vi "UDP Data Link - Action VIs - ActionVIOnSave.vi"(8 "error in (no error)":errorcluster, 11 "Device Item Ref in":T1 format="%.0x") -> (0 "error out":errorcluster, 3 "Device Item Ref out":T1 format="%.0x")   [LabVIEW 2015, in "UDP-Custom-Device System Explorer.lvlib"]
uses:
  UDP-Custom-Device System Explorer.lvlib
  <vilib>/NI Veristand/Custom Device API/Custom Device Item Ref.ctl
  Shared/Constants.vi
  <vilib>/NI Veristand/Custom Device API/Get Item Property (Boolean).vi
  <vilib>/NI Veristand/Custom Device API/Get Item Property (Path).vi
  <vilib>/NI VeriStand/Custom Device API/Custom Device API.lvlib
  Shared/UDP-Custom-Device Shared.lvlib
  <vilib>/NI VeriStand/Custom Device Tools/Custom Device Utility Library/Custom Device Utility Library.lvlib
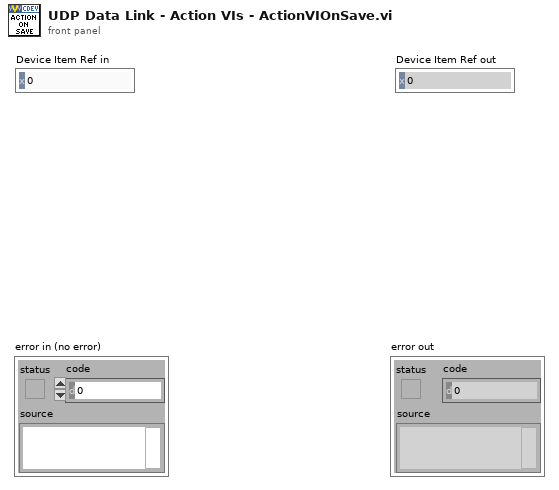
[diagram p1: front panel]
types:
  T1 = typedef "Custom Device API.lvlib/Custom Device Item Ref.ctl" = u64
  T2 = typedef "UDP-Custom-Device System Explorer.lvlib/UDP Data Link - TypeDefs - XML Header Data.ctl" = cluster{"Revision (\"Major.Minor.Fix.Build\")":string, "Creation Date (\"yyyy-mm-dd\")":string, "Controller Name":string}
  T3 = typedef "UDP-Custom-Device System Explorer.lvlib/UDP Data Link - TypeDefs - XML Group.ctl" = cluster{"Freq":i32, "Tx Channels":T4[], "Rx Channels":T4[]}
  T4 = typedef "UDP-Custom-Device System Explorer.lvlib/UDP Data Link - TypeDefs - XML Channel.ctl" = cluster{"Channel Name":string, "Data Type":u16, "Description":string, "Unit":string}
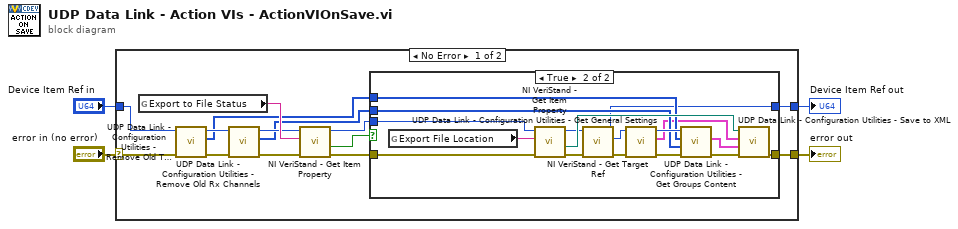
[diagram p0: block diagram]
diagram:
  n1 = case shown="No Error" "error in (no error)" {
    selector: "error in (no error)" -> [w17 w39]
    tunnel: [w6 w39] -> w3
    tunnel: "Device Item Ref in" -> [w18 w38]
    tunnel: [w5 w38] -> w1
    frame No Error {
      n2 = global read "Constants.vi" "Export to File Status"() -> (w14:string)
      n3 = call "UDP Data Link - Configuration Utilities - Remove Old Tx Channels.vi"("error in (no error)"=w17, "Device Item Ref in"=w18) -> ("error out"=w16:errorcluster, "Tx Dependent Refs"=w8:T1[], "Device Item Ref out"=w15:T1)  [unwired: 7 in]
      n4 = call "UDP Data Link - Configuration Utilities - Remove Old Rx Channels.vi"("error in (no error)"=w16, "Device Item Ref in"=w15) -> ("error out"=w12:errorcluster, "Rx Dependent Refs"=w7:T1[], "Device Item Ref out"=w13:T1)  [unwired: 7 in]
      n5 = call-poly <vilib>:"NI VeriStand - Get Item Property.vi"("error in (no error)"=w12, "Property Name"=w14, "Item Ref in"=w13) -> ("error out"=w10:errorcluster, "Value"=w11:bool, "Item Ref out"=w9:T1)  [unwired: 5 in, 1 out]
      n6 = case shown="True" w11 {
        tunnel: w10 -> [w20 w37]
        tunnel: w9 -> [w19 w36]
        tunnel: w8 -> [_ w28]
        tunnel: w7 -> [_ w27]
        tunnel: [w20 w22] -> w6
        tunnel: [w19 w21] -> w5
        frame False {
        }
        frame True {
          n7 = global read "Constants.vi" "Export File Location"() -> (w35:string)
          n8 = call-poly <vilib>:"NI VeriStand - Get Item Property.vi"("error in (no error)"=w37, "Property Name"=w35, "Item Ref in"=w36) -> ("error out"=w33:errorcluster, "Value"=w34:path, "Item Ref out"=w32:T1)  [unwired: 5 in, 1 out]
          n9 = call <vilib>:"NI VeriStand - Get Target Ref.vi"("error in"=w33, "Item Ref in"=w32) -> ("error out"=w30:errorcluster, "Target Ref"=w31:T1, "Item Ref out"=w21:T1)  [unwired: 6 in, 1 out]
          n10 = call "UDP Data Link - Configuration Utilities - Get General Settings.vi"("error in (no error)"=w30, "Target Ref in"=w31) -> ("error out"=w26:errorcluster, "XML Header Data"=w24:T2, "Target Ref out"=w29:T1)  [unwired: 7 in]
          n11 = call "UDP Data Link - Configuration Utilities - Get Groups Content.vi"("error in (no error)"=w26, "Rx"=w27, "Tx"=w28, "Target Ref In"=w29) -> ("error IO"=w25:errorcluster, "Groups"=w23:T3[])  [unwired: 5 in, 1 out]
          n12 = call "UDP Data Link - Configuration Utilities - Save to XML.vi"("error in"=w25, "Channel Groups"=w23, "XML Header Data"=w24, "XML File Path"=w34) -> ("error out"=w22:errorcluster)  [unwired: 7 in]
        }
      }
    }
    frame Error {
    }
  }
  "error out" <- w3
  "Device Item Ref out" <- w1
